vi "Check Home Position Part 1.vi"(8 "error in (no error)":errorcluster, 9 "Amphipods in":refnum<class "Amphipod.lvclass">[](array[class]), 10 "Home":i8, 11 "Position in":cluster{"Row":i8, "Column":i8}) -> (0 "error out":errorcluster, 2 "Position out":cluster{"Row":i8, "Column":i8}[](array[cluster]), 3 "Column":i8)   [LabVIEW 2019, in "23.lvlib" / "Amphipod.lvclass"]
uses:
  Amphipod.lvclass
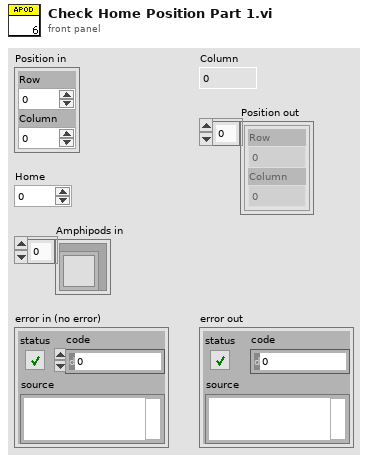
[diagram p1: front panel]
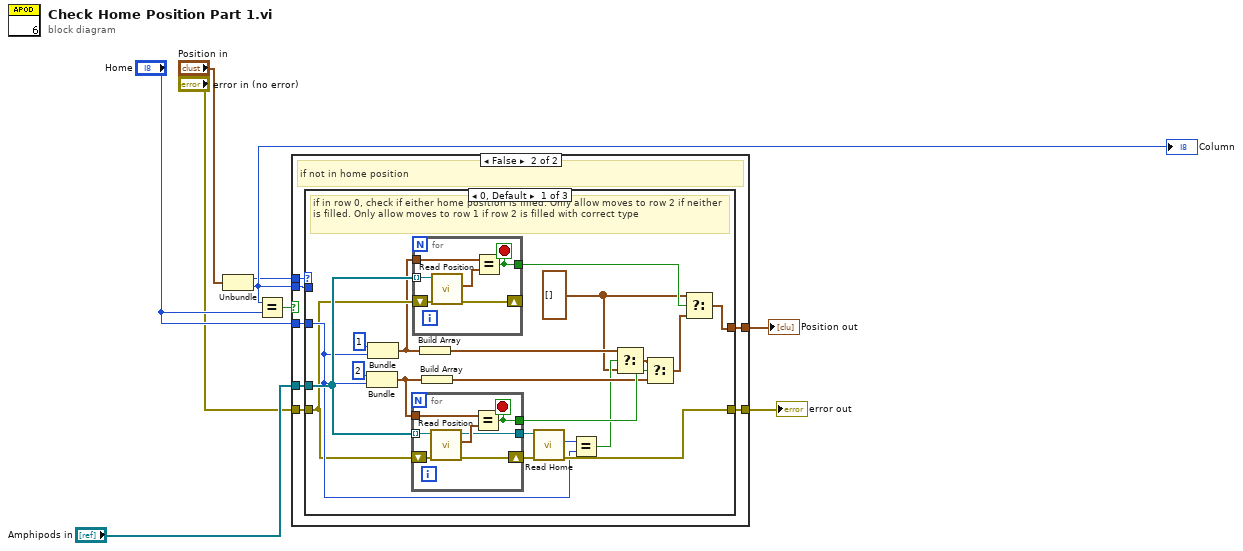
[diagram p0: block diagram]
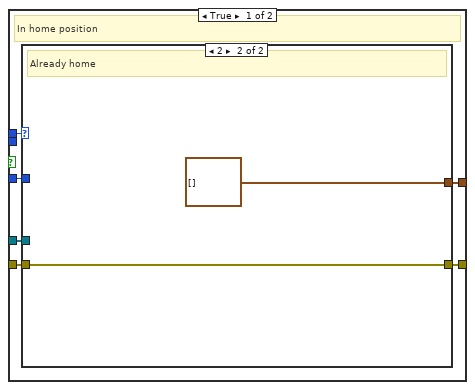
[diagram p2: hidden frame]
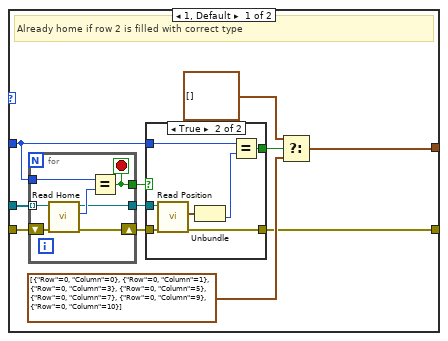
[diagram p3: hidden frame]
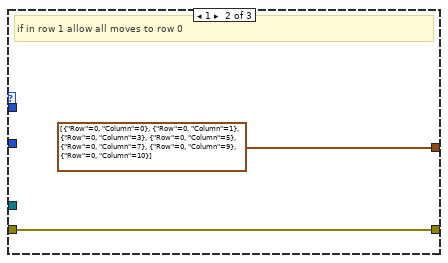
[diagram p5: hidden frame]
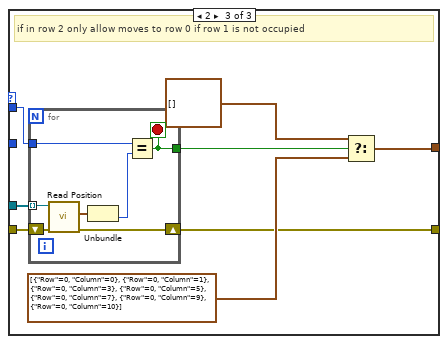
[diagram p6: hidden frame]
diagram:
  n1 = Unbundle("Position in") -> ("Row"=w2:i8, "Column"=w9:i8)
  "Column" <- w9
  n2 = Equal?(x=w9, y="Home") -> (x = y?=w1:bool)
  n3 = case shown="False" w1 {
    tunnel: "Amphipods in" -> [w14 w49]
    tunnel: w2 -> [w15 w50]
    tunnel: "Home" -> [w13 w48]
    tunnel: [w12 w47] -> w5
    tunnel: "error in (no error)" -> [w11 w46]
    tunnel: [w10 w45] -> w8
    tunnel: w9 -> [_ w44]
    frame True {
      # "In home position"
      n4 = case shown="2" w15 {
        tunnel: w14 -> [w26 _]
        tunnel: w13 -> [w17 _]
        tunnel: [w22 cluster{"Row":i8, "Column":i8}[] [] ("t")] -> w12
        tunnel: w11 -> [w21 w42]
        tunnel: [w19 w42] -> w10
        frame 1, Default {
          # "Already home if row 2 is filled with correct type"
          n5 = for {
            tunnel: w26 -> [w41] mode=indexing
            tunnel: w17 -> [w39]
            tunnel: [w38] -> w25
            shift-right: [w36] -> w20
            shift-left: w21 -> [w37]
            tunnel: [w35] -> w18
            stop <- w35 stop-if-true
            n6 = call-dynamic "Read Home.vi"("error in (no error)"=w37, "Amphipod in"=w41) -> ("error out"=w36:errorcluster, "Home"=w40:i8, "Amphipod out"=w38:refnum<class "Amphipod.lvclass">)  [unwired: 7 in]
            n7 = Equal?(x=w39, y=w40) -> (x = y?=w35:bool)
          }
          n8 = case shown="True" w18 {
            tunnel: w25 -> [_ w34]
            tunnel: w20 -> [w27 w32]
            tunnel: [w27 w31] -> w19
            tunnel: w17 -> [_ w28]
            tunnel: [_ w29] -> w16
            frame False {
            }
            frame True {
              n9 = call-dynamic "Read Position.vi"("error in (no error)"=w32, "Amphipod in"=w34) -> ("error out"=w31:errorcluster, "Position"=w33:cluster{"Row":i8, "Column":i8})  [unwired: 7 in, 1 out]
              n10 = Unbundle(w33) -> ("Column"=w30:i8)  [unwired: 1 out]
              n11 = Equal?(x=w28, y=w30) -> (x = y?=w29:bool)
            }
          }
          n12 = Select(t=cluster{"Row":i8, "Column":i8}[] [], s=w16, f=cluster{"Row":i8, "Column":i8}[] [{"Row"=0, "Column"=0}, {"Row"=0, "Column"=1}, {"Row"=0, "Column"=3}, {"Row"=0, "Column"=5}, {"Row"=0, "Column"=7}, {"Row"=0, "Column"=9}, {"Row"=0, "Column"=10}] ("Position")) -> (s? t:f=w22:cluster{"Row":i8, "Column":i8}[])
        }
        frame 2 {
          # "Already home"
        }
      }
    }
    frame False {
      # "if not in home position"
      n13 = case shown="0, Default" w50 {
        tunnel: w49 -> [w68 _ w93]
        tunnel: w48 -> [w61 _ _]
        tunnel: [w66 cluster{"Row":i8, "Column":i8}[] [{"Row"=0, "Column"=0}, {"Row"=0, "Column"=1}, {"Row"=0, "Column"=3}, {"Row"=0, "Column"=5}, {"Row"=0, "Column"=7}, {"Row"=0, "Column"=9}, {"Row"=0, "Column"=10}] ("Position") w90] -> w47
        tunnel: w46 -> [w59 w85 w89]
        tunnel: [w63 w85 w87] -> w45
        tunnel: w44 -> [_ _ w86]
        frame 0, Default {
          w51 = cluster{"Row":i8, "Column":i8}[] [] ("t")
          # "if in row 0, check if either home position is filled. Only allow moves to row 2 if neither is filled. Only allow moves to row 1 if row 2 is filled with correct type"
          n14 = Bundle("Row"=i8 2, "Home"=w61) -> (w56:cluster{"Row":i8, "Home":i8})  [unwired: 1 in]
          n15 = Bundle("Row"=i8 1, "Home"=w61) -> (w58:cluster{"Row":i8, "Home":i8})  [unwired: 1 in]
          n16 = for {
            tunnel: w68 -> [w83] mode=indexing
            tunnel: w56 -> [w80]
            shift-right: [w78] -> w64
            shift-left: w59 -> [w82]
            tunnel: [w79] -> w60
            tunnel: [w77] -> w65
            stop <- w79 stop-if-true
            n17 = call-dynamic "Read Position.vi"("error in (no error)"=w82, "Amphipod in"=w83) -> ("error out"=w78:errorcluster, "Position"=w81:cluster{"Row":i8, "Column":i8}, "Amphipod out"=w77:refnum<class "Amphipod.lvclass">)  [unwired: 7 in]
            n18 = Equal?(x=w80, y=w81) -> (x = y?=w79:bool)
          }
          n19 = for {
            tunnel: w68 -> [w71] mode=indexing
            tunnel: w58 -> [w74]
            shift-right: [w73] -> _
            shift-left: w59 -> [w76]
            tunnel: [w72] -> w67
            stop <- w72 stop-if-true
            n20 = call-dynamic "Read Position.vi"("error in (no error)"=w76, "Amphipod in"=w71) -> ("error out"=w73:errorcluster, "Position"=w75:cluster{"Row":i8, "Column":i8})  [unwired: 7 in, 1 out]
            n21 = Equal?(x=w74, y=w75) -> (x = y?=w72:bool)
          }
          n22 = Build Array(w58) -> (w52:cluster{"Row":i8, "Home":i8}[])
          n23 = Build Array(w56) -> (w55:cluster{"Row":i8, "Home":i8}[])
          n24 = call-dynamic "Read Home.vi"("error in (no error)"=w64, "Amphipod in"=w65) -> ("error out"=w63:errorcluster, "Home"=w62:i8)  [unwired: 7 in, 1 out]
          n25 = Equal?(x=w62, y=w61) -> (x = y?=w54:bool)
          n26 = Select(t=w52, s=w54, f=w51) -> (s? t:f=w53:cluster{"Row":i8, "Column":i8}[])
          n27 = Select(t=w53, s=w60, f=w55) -> (s? t:f=w57:cluster{"Row":i8, "Home":i8}[])
          n28 = Select(t=w51, s=w67, f=w57) -> (s? t:f=w66:cluster{"Row":i8, "Home":i8}[])
        }
        frame 1 {
          # "if in row 1 allow all moves to row 0"
        }
        frame 2 {
          # "if in row 2 only allow moves to row 0 if row 1 is not occupied"
          n29 = for {
            tunnel: w93 -> [w99] mode=indexing
            tunnel: w86 -> [w100]
            shift-right: [w95] -> w87
            shift-left: w89 -> [w98]
            tunnel: [w94] -> w88
            stop <- w94 stop-if-true
            n30 = call-dynamic "Read Position.vi"("error in (no error)"=w98, "Amphipod in"=w99) -> ("error out"=w95:errorcluster, "Position"=w97:cluster{"Row":i8, "Column":i8})  [unwired: 7 in, 1 out]
            n31 = Unbundle(w97) -> ("Column"=w96:i8)  [unwired: 1 out]
            n32 = Equal?(x=w100, y=w96) -> (x = y?=w94:bool)
          }
          n33 = Select(t=cluster{"Row":i8, "Column":i8}[] [], s=w88, f=cluster{"Row":i8, "Column":i8}[] [{"Row"=0, "Column"=0}, {"Row"=0, "Column"=1}, {"Row"=0, "Column"=3}, {"Row"=0, "Column"=5}, {"Row"=0, "Column"=7}, {"Row"=0, "Column"=9}, {"Row"=0, "Column"=10}] ("Position")) -> (s? t:f=w90:cluster{"Row":i8, "Column":i8}[])
        }
      }
    }
  }
  "error out" <- w8
  "Position out" <- w5
